vi "PH_Periodic_Sequencer.PC PPStatePU.vi"(0 "i ref in":refnum<vi>, 2 "Service Name":string, 3 "State":T1 items=["no info", "off/false/out", "on/true/in", "Failure", "Alarm", "Status 1", "Status 2", "Status 3"], 4 "not linked?":bool, 5 "error in (no error)":errorcluster) -> (14 "i ref out":refnum<vi>, 19 "error out":errorcluster)   [LabVIEW 2014, in "PH_Periodic_Sequencer.lvlib"]
doc: "This VI writes the state of the PU to own attributes and the GUI elements."
uses:
  PH_Periodic_Sequencer.lvlib
  PH_StatusHandler/PH_StatusHandler.Status.ctl
  PH_StatusHandler/PH_StatusHandler.lvlib
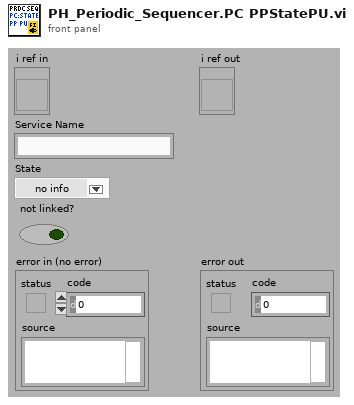
[diagram p1: front panel]
types:
  T1 = typedef "PH_StatusHandler.lvlib/PH_StatusHandler.Status.ctl" = i16
  T2 = typedef "PH_Periodic_Sequencer.lvlib/PH_Periodic_Sequencer.i attribute.ctl" = cluster{"GUI Refs":cluster{"Main Off":refnum<vi>, "Start":refnum<vi>, "Ready":refnum<vi>, "Sequencer SM State":refnum<vi>, "Interval [sec]":refnum<vi>, "Wanted Shots":refnum<vi>, "Delivered Shots":refnum<vi>}, "PU Info":cluster{"Instancename":string, "State":T1, "linked":bool}[], "Sequencer":cluster{"Instancename":string, "linked?":bool, "R2S?":bool, "SM State":string}, "Run?":bool, "Interval [sec]":dbl, "PU State Refs":refnum<vi>[], "Wanted Shots":i32, "Delivered Shots":i32}
  T3 = cluster{"Instancename":string, "State":T1, "linked":bool}[]
  T4 = cluster{"Instancename":string, "State":T1, "linked":bool}
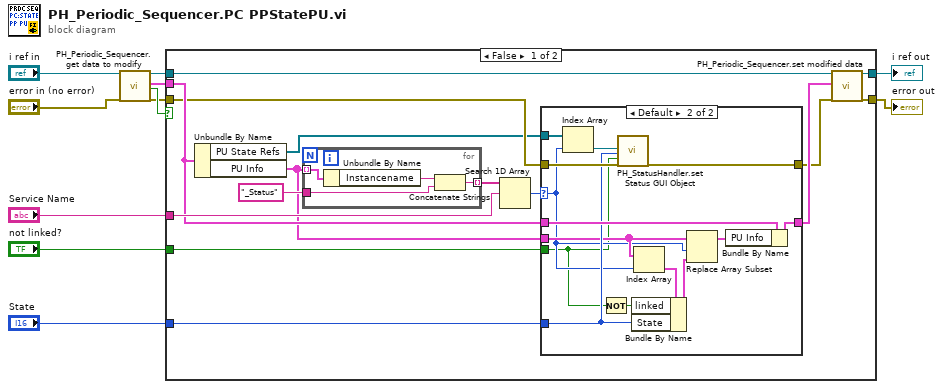
[diagram p0: block diagram]
diagram:
  n1 = call "PH_Periodic_Sequencer.get data to modify.vi"("i ref in"="i ref in", "error in (no error)"="error in (no error)") -> ("i ref out"=w4:refnum<vi>, "i attribute"=w8:T2, "timed out"=w11:bool, "error out"=w6:errorcluster)  [unwired: 14 in]
  n2 = case shown="False" w11 {
    tunnel: w4 -> [w26 w48]
    tunnel: [w25 w48] -> w5
    tunnel: w6 -> [w15 w47]
    tunnel: [w24 w47] -> w7
    tunnel: w8 -> [w19 _]
    tunnel: "State" -> [w22 _]
    tunnel: "Service Name" -> [w21 _]
    tunnel: "not linked?" -> [w14 _]
    frame False {
      n3 = Unbundle By Name(w19) -> ("PU State Refs"=w12:refnum<vi>[], "PU Info"=w13:T3)
      n4 = for {
        tunnel: w13 -> [w30] mode=indexing
        tunnel: "_Status" -> [w28]
        tunnel: [w27] -> w17 mode=indexing
        n5 = Unbundle By Name(w30) -> ("Instancename"=w29:string)
        n6 = Concatenate Strings(w29, w28) -> (w27:string)
      }
      n7 = Search 1D Array(1D array=w17, element=w21) -> (index of element=w20:i32)  [unwired: 1 in]
      n8 = case shown="Default" w20 {
        selector: w20 -> [_ w35]
        tunnel: [w32 w46] -> w23
        tunnel: w19 -> [w32 w45]
        tunnel: w22 -> [_ w39]
        tunnel: w12 -> [_ w44]
        tunnel: [w31 w42] -> w16
        tunnel: w15 -> [w31 w41]
        tunnel: w14 -> [_ w33]
        tunnel: w13 -> [_ w38]
        frame -1 {
        }
        frame Default {
          n9 = Index Array(array=w44, index=w35) -> (element=w43:refnum<vi>)
          n10 = Not(x=w33) -> (.not. x?=w34:bool)
          n11 = call "PH_StatusHandler.set Status GUI Object.vi"("PH Status Ref"=w43, "Value"=w39, "Blinking (false)"=w33, "error in (no error)"=w41) -> ("error out"=w42:errorcluster)  [unwired: 15 in]
          n12 = Index Array(array=w38, index=w35) -> (element=w40:T4)
          n13 = Bundle By Name(cluster=w40, "linked"=w34, "State"=w39) -> (w37:T4)
          n14 = Replace Array Subset(array=w38, new element=w37, index=w35) -> (w36:T3)
          n15 = Bundle By Name(cluster=w45, "PU Info"=w36) -> (w46:T2)
        }
      }
      n16 = call "PH_Periodic_Sequencer.set modified data.vi"("i ref in"=w26, "i attribute"=w23, "error in (no error)"=w16) -> ("i ref out"=w25:refnum<vi>, "error out"=w24:errorcluster)  [unwired: 15 in]
    }
    frame True {
    }
  }
  "error out" <- w7
  "i ref out" <- w5
